vi "Eval.Mathematica.vi"(0 "input":string, 1 "reference":refnum<k24>) -> ()   [LabVIEW 2014]
uses:
  D:/Projects/pylua/LabVIEW/Wolfram.NETLink.dll
  Wolfram.NETLink.dll
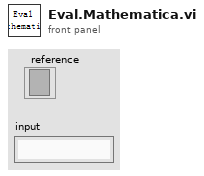
[diagram p1: front panel]
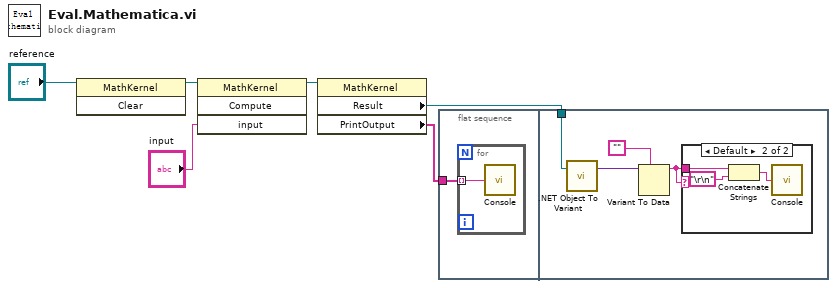
[diagram p0: block diagram]
diagram:
  n1 = invoke class="MathKernel" method="Clear"(reference="reference") -> (reference out=w6:refnum<k24>)  [unwired: 2 in, 2 out]
  n2 = invoke class="MathKernel" method="Compute"(reference=w6, "input"="input") -> (reference out=w5:refnum<k24>)  [unwired: 2 in, 3 out]
  n3 = property class="MathKernel"(reference=w5) -> ("Result"=w4:refnum<k24>, "PrintOutput"=w3:string[])  [unwired: 1 in, 2 out]
  n4 = flat-sequence {
    tunnel: w3 -> [w7]
    tunnel: w4 -> [w9]
    frame #0 {
      n5 = for {
        tunnel: w7 -> [w8] mode=indexing
        n6 = call "Console.vi"("print string"=w8) -> ()  [unwired: 1 in]
      }
    }
    frame #1 {
      n7 = call <vilib>:".NET Object To Variant.vi"(".NET object"=w9) -> ("variant"=w11:variant)  [unwired: 1 in, 1 out]
      n8 = Variant To Data(type="", Variant=w11) -> (data=w12:string)  [unwired: 1 in, 1 out]
      n9 = case shown="Default" w12 {
        tunnel: w12 -> [_ w14]
        frame "Null" {
        }
        frame Default {
          n10 = Concatenate Strings(w14, "\r\n") -> (w13:string)
          n11 = call "Console.vi"("print string"=w13) -> ()  [unwired: 1 in]
        }
      }
    }
  }
